vi "Execution End.vi"(8 "error in (no error)":errorcluster, 11 "Execution in":refnum<data-value>) -> (0 "error out":errorcluster, 3 "Execution out":refnum<data-value>)   [LabVIEW 2015, in "Execution.lvclass"]
uses:
  Execution.lvclass
  EXECUTION_STATUS.ctl
  EXECUTION_UI_MSG.ctl
  Send UI Message.vi
  Step.lvclass
  Project.lvclass
  Plugin.lvclass
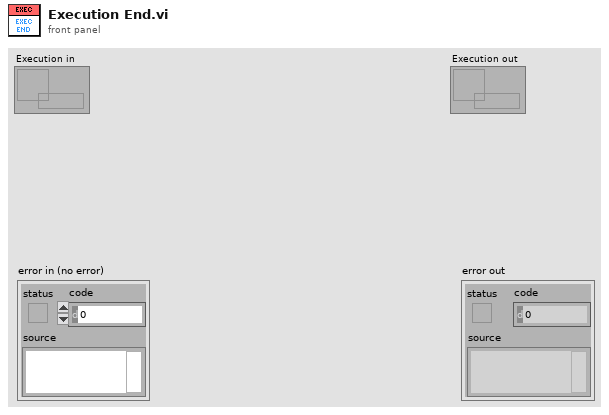
[diagram p1: front panel]
types:
  T1 = typedef "Execution.lvclass/EXECUTION_UI_MSG.ctl" = enum16{"EXECUTION_STATUS", "INIT_UI", "DUT_UPDATE", "BOTTOM_PANEL_UPDATE", "TOP_PANEL_UPDATE", "STEP_START", "STEP_END", "DISPLAY_RESULT", "APPLICATION_END"}
  T2 = typedef "Execution.lvclass/EXECUTION_STATUS.ctl" = enum16{"Initializing ", "Disable", "Ready", "Running", "Finished"}
  T3 = typedef "Execution.lvclass/EXECUTION_RESULT_TYPEDEF.ctl" = enum16{"Unknow", "Terminated", "Passed", "Failed", "Error"}
  T4 = typedef "Execution.lvclass/EXECUTION_CONTEXT.ctl" = cluster{"Continue Test":bool, "DUT Info":T5, "StartTime":timestamp, "EndTime":timestamp, "Result":T3, "Info Text":string, "ResultList":T6[]}
  T5 = typedef "Execution.lvclass/DUT_INFO_TYPEDEF.ctl" = cluster{"SN":string, "Model":string, "PartNumber":string, "Revision":string, "Software":string, "Hardware":string}
  T6 = typedef "Execution.lvclass/STEP_RESULT.ctl" = cluster{"StepIndex":u32, "Step":refnum<class "Step.lvclass">, "StartTime":timestamp, "EndTime":timestamp, "Result":T7, "Error Info":string, "Measure Results":T8[]}
  T7 = typedef "Step.lvclass/STEP_STATUS.ctl" = enum16{"Skipped", "Done", "Passed", "Failed", "Error"}
  T8 = typedef "Execution.lvclass/STEP_MEASURE_RESULT.ctl" = cluster{"Name":string, "Data Type":T9, "Check Type":T10, "String Limit":string, "Lower Limit":dbl, "Upper Limit":dbl, "Boolean Limit":bool, "Ignore Case":bool, "Measure Data":variant, "Result":T7, "Error Info":string}
  T9 = typedef "Step.lvclass/OUTPUT_DATA_TYPE.ctl" = enum16{"Boolean", "String", "Numeric", "Other"}
  T10 = typedef "Step.lvclass/OUTPUT_CHECK_TYPE.ctl" = enum16{"INVALID", "DO_NOT_CHECK", "RECORD", "VARIABLE", "EQUAL", "NOT_EQUAL", "STR_CONTAINS", "STR_START_WITH", "STR_END_WITH", "STR_REGEX_MATCH", "NUM_GT", "NUM_LT", "NUM_GE", "NUM_LE", "NUM_RANGE", "NUM_RANGE_BDY"}
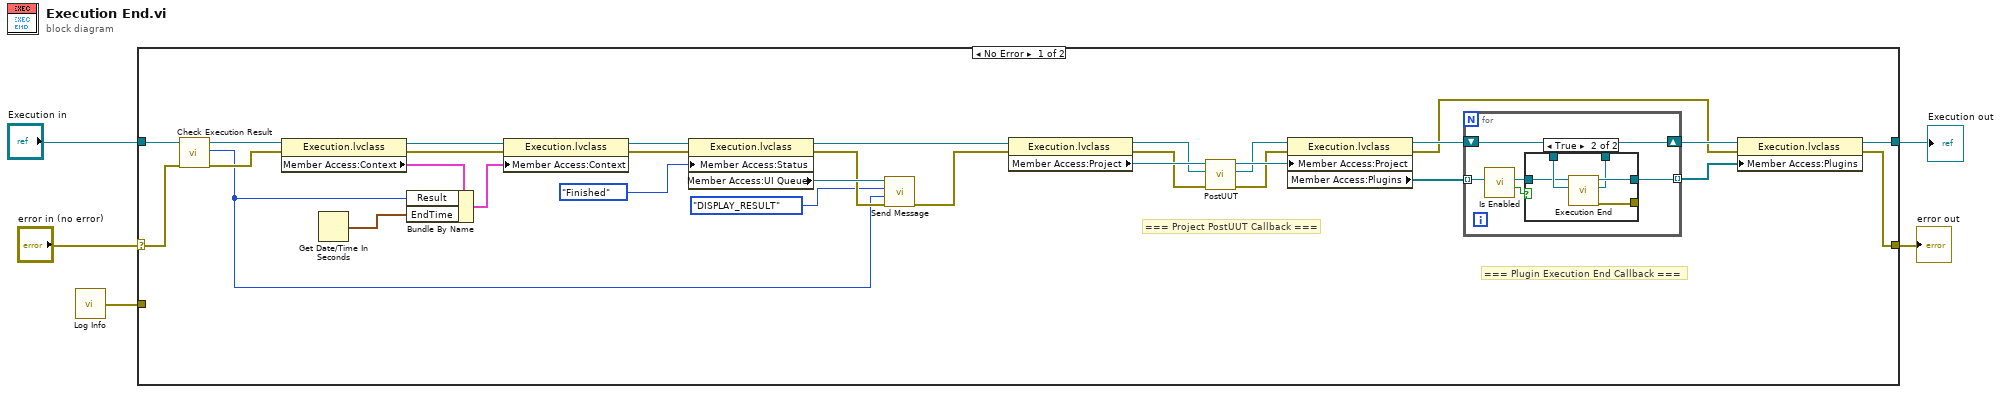
[diagram p0: block diagram]
diagram:
  n1 = call "Log Info.vi"() -> ("error out"=w1:errorcluster)  [unwired: 5 in]
  n2 = case shown="No Error" "error in (no error)" {
    selector: "error in (no error)" -> [w17 w51]
    tunnel: [w14 w51] -> w4
    tunnel: [w15 w50] -> w3
    tunnel: "Execution in" -> [w19 w50]
    tunnel: w1 -> [_ _]
    frame No Error {
      # "=== Plugin Execution End Callback ==="
      # "=== Project PostUUT Callback ==="
      n3 = call "Check Execution Result.vi"("error in (no error)"=w17, "Execution in"=w19) -> ("error out"=w16:errorcluster, "Execution Result"=w7:T3, "Execution out"=w18:refnum<data-value>)  [unwired: 7 in]
      n4 = property class="Execution.lvclass"(reference=w18, error in=w16) -> (reference out=w24:refnum<data-value>, error out=w23:errorcluster, "Member Access:Context"=w21:T4)
      n5 = Get Date/Time In Seconds() -> (seconds since 1Jan1904=w22:timestamp)
      n6 = Bundle By Name(cluster=w21, "Result"=w7, "EndTime"=w22) -> (w20:T4)
      n7 = property class="Execution.lvclass"(reference=w24, error in=w23, "Member Access:Context"=w20) -> (reference out=w13:refnum<data-value>, error out=w12:errorcluster)
      n8 = property class="Execution.lvclass"(reference=w13, error in=w12, "Member Access:Status"=EXECUTION_STATUS."Finished" ("Status")) -> (reference out=w11:refnum<data-value>, error out=w9:errorcluster, "Member Access:UI Queue"=w10:refnum<queue>)
      n9 = call-poly "Send Message.vi"("error in (no error)"=w9, "Data"=w7, "Msg"=EXECUTION_UI_MSG."DISPLAY_RESULT", "UI Queue"=w10) -> ("error out"=w6:errorcluster)  [unwired: 7 in]
      n10 = property class="Execution.lvclass"(reference=w11, error in=w6) -> (reference out=w26:refnum<data-value>, error out=w34:errorcluster, "Member Access:Project"=w35:refnum<class "Project.lvclass">)
      n11 = call-dynamic "PostUUT.vi"("error in (no error)"=w34, "Execution in"=w26, "TestProjectBase in"=w35) -> ("error out"=w32:errorcluster, "Execution out"=w25:refnum<data-value>, "TestProjectBase out"=w33:refnum<class "Project.lvclass">)  [unwired: 6 in]
      n12 = property class="Execution.lvclass"(reference=w25, error in=w32, "Member Access:Project"=w33) -> (reference out=w31:refnum<data-value>, error out=w27:errorcluster, "Member Access:Plugins"=w30:refnum<class "Plugin.lvclass">[])
      n13 = for {
        shift-right: [w40] -> w29
        shift-left: w31 -> [w41]
        tunnel: w30 -> [w39] mode=indexing
        tunnel: [w42] -> w28 mode=indexing
        n14 = call "Is Enabled.vi"("Plugin in"=w39) -> ("Enabled"=w37:bool, "Plugin out"=w38:refnum<class "Plugin.lvclass">)  [unwired: 9 in]
        n15 = case shown="True" w37 {
          tunnel: [w44 w49] -> w42
          tunnel: [_ w48] -> _
          tunnel: w41 -> [w43 w47]
          tunnel: [w43 w46] -> w40
          tunnel: w38 -> [w44 w45]
          frame False {
          }
          frame True {
            n16 = call-dynamic "Execution End.vi"("Execution in"=w47, "Plugin in"=w45) -> ("error out"=w48:errorcluster, "Execution out"=w46:refnum<data-value>, "Plugin out"=w49:refnum<class "Plugin.lvclass">)  [unwired: 7 in]
          }
        }
      }
      n17 = property class="Execution.lvclass"(reference=w29, error in=w27, "Member Access:Plugins"=w28) -> (reference out=w15:refnum<data-value>, error out=w14:errorcluster)
    }
    frame Error {
    }
  }
  "error out" <- w4
  "Execution out" <- w3
